vi "Cryo Sep Front Panel.vi"() -> ()   [LabVIEW 2019, in "Results.lvlib" / "Cryo Sep Results.lvclass"]
uses:
  Cryo Sep Results.lvclass
  Test Stands/Cryo Sep/Cryo Sep Test Stand.lvclass
panel:
  out "Temp Timeprofiles":waveform(dbl)[](graph) caption="Temperatures"
  out "Tc5":dbl(slide) scale=0.0..100.0
  out "Tc6":dbl(slide) scale=0.0..100.0
  out "Tc7":dbl(slide) scale=0.0..100.0
  out "Tc8":dbl(slide) scale=0.0..100.0
  out "Tc9":dbl(slide) scale=0.0..100.0
  out "Tc10":dbl(slide) scale=0.0..100.0
  out "Tc11":dbl(slide) scale=0.0..100.0
  out "Tc12":dbl(slide) scale=0.0..100.0
  out "Tc4":dbl(slide) scale=0.0..100.0
  out "Tc4A":dbl(slide) scale=0.0..100.0
  out "Tc4B":dbl(slide) scale=0.0..100.0
  out "Tc4C":dbl(slide) scale=0.0..100.0
  out "Tc2":dbl(slide) scale=0.0..100.0
  out "Tc3":dbl(slide) scale=0.0..100.0
  out "Tc1":dbl(slide) scale=0.0..100.0
  out "Tc0":dbl(slide) max=100.0 scale=0.0..100.0
  out "Tin1":dbl(slide) scale=0.0..100.0
  out "Pressure (abs)":dbl format="%#.2f"
  out "Flow":dbl format="%#.2f"
  out "Tin0":dbl(slide) scale=0.0..100.0
  # "Cryogenic Separator"
  # "l/min (n)"
  # "bar"
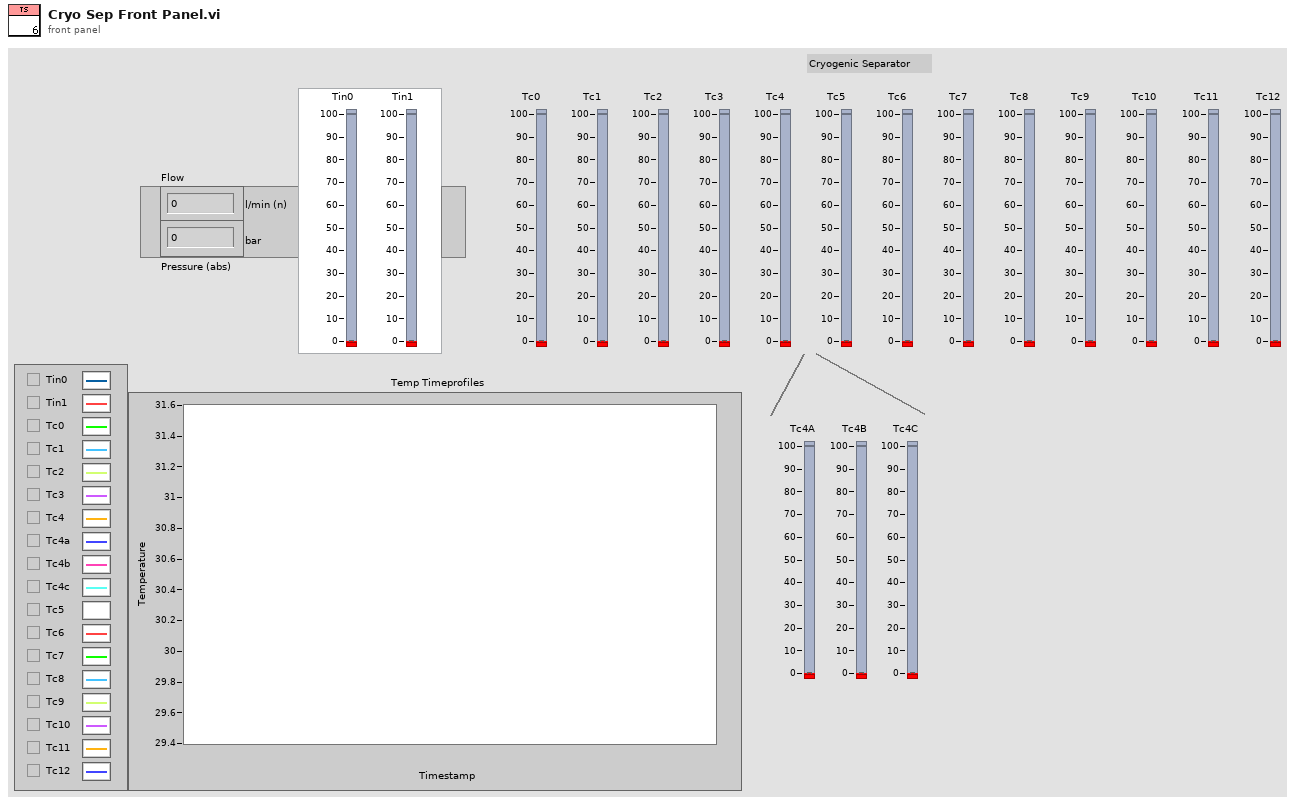
[diagram p1: front panel]
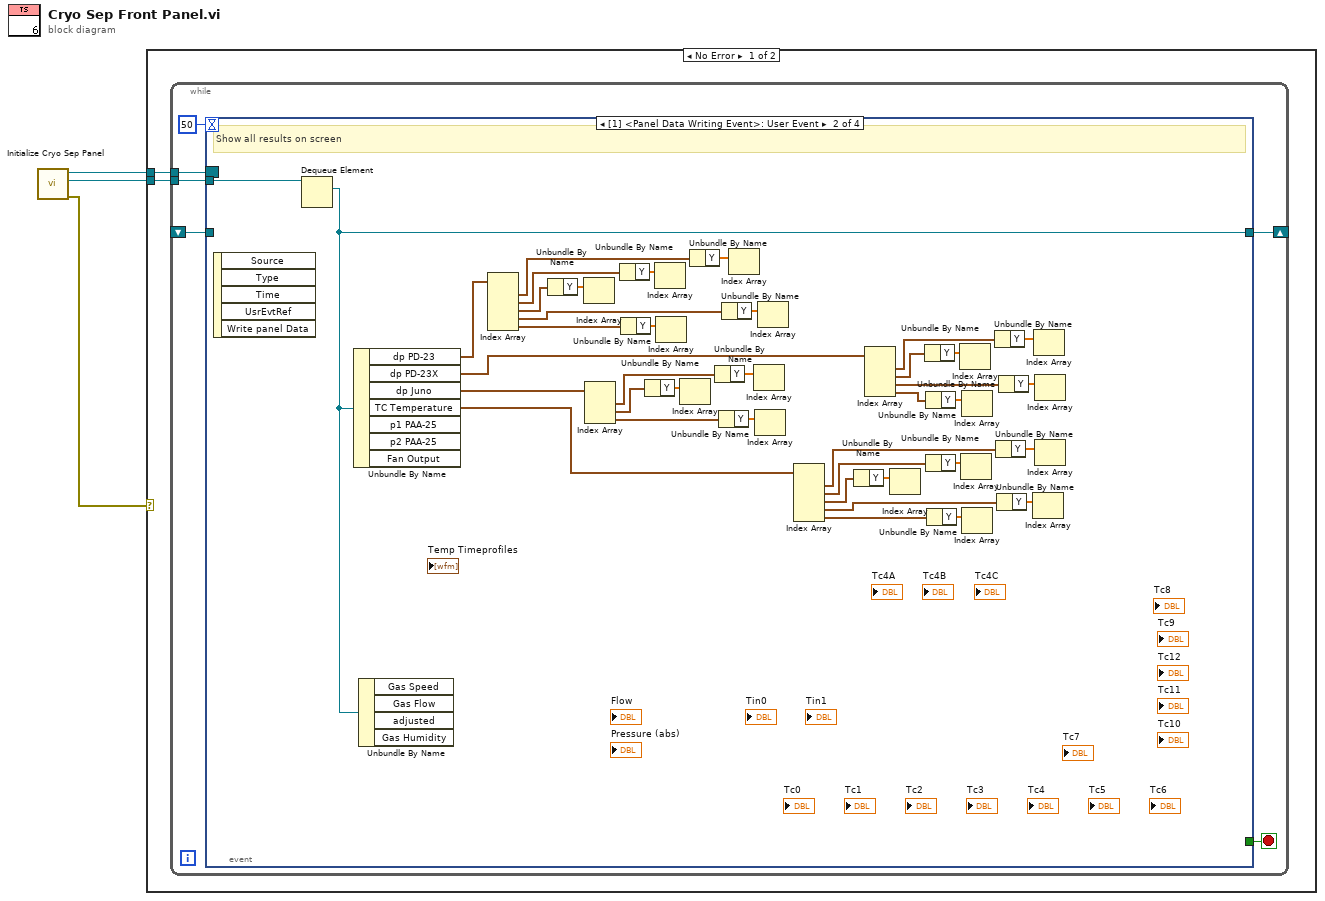
[diagram p0: block diagram]
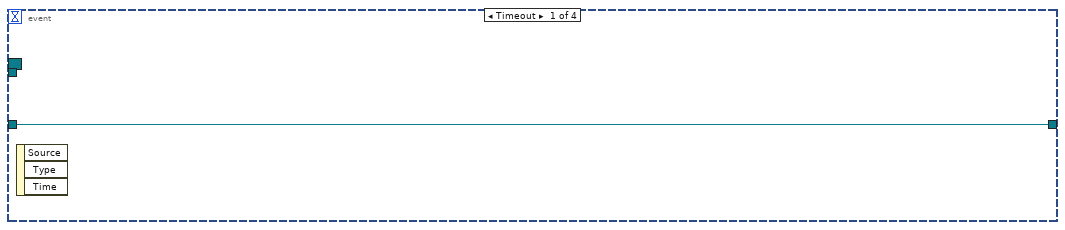
[diagram p2: hidden frame]
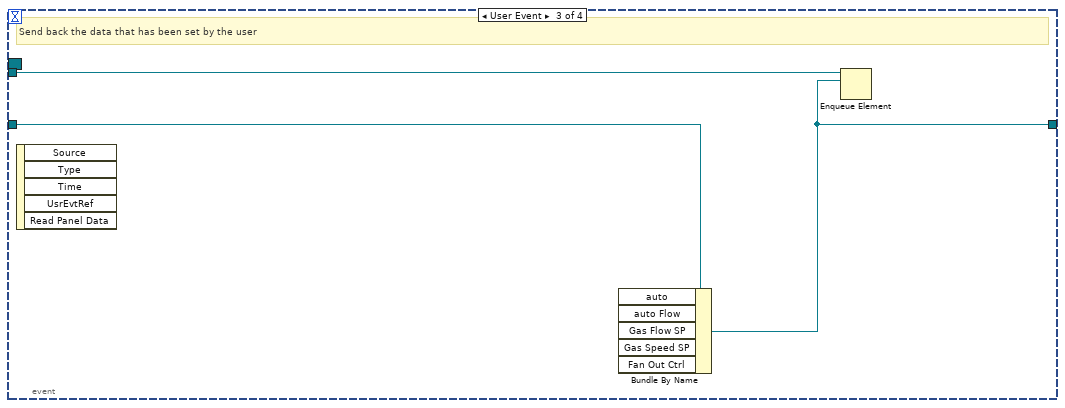
[diagram p3: hidden frame]
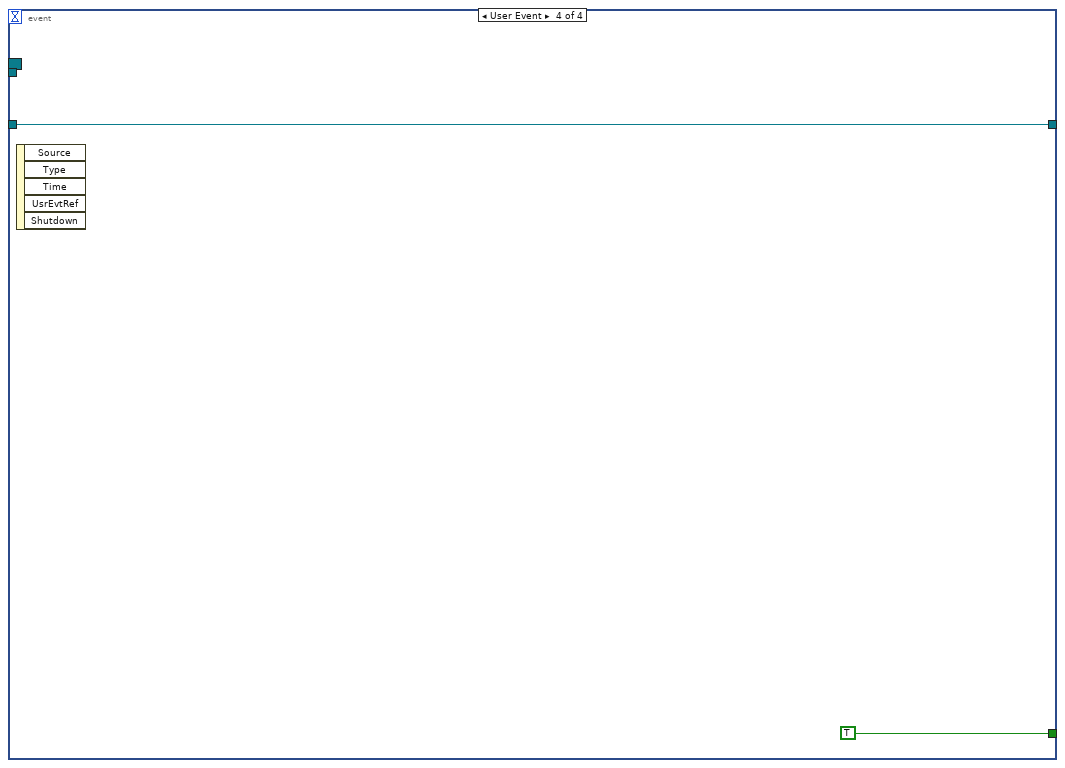
[diagram p4: hidden frame]
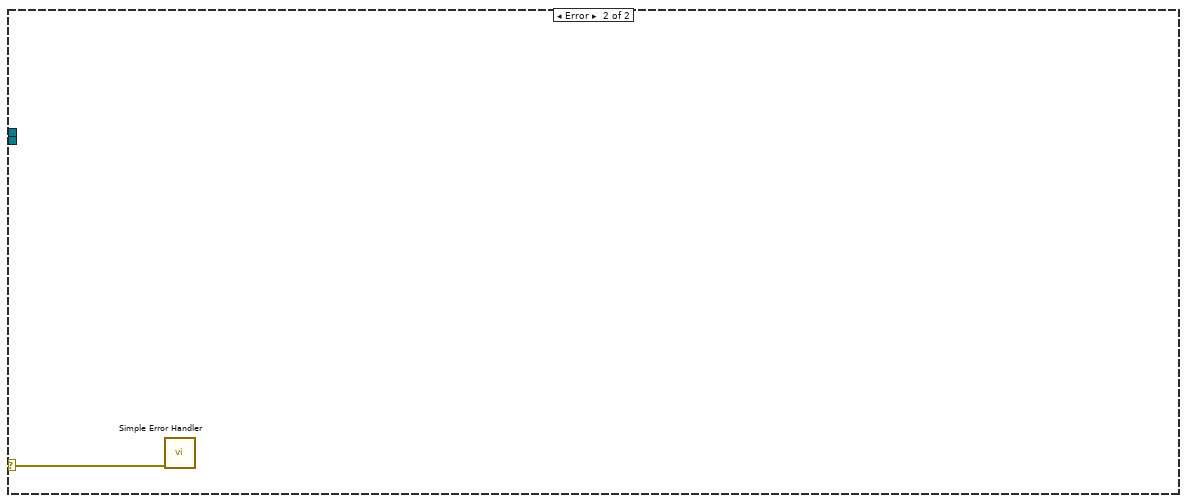
[diagram p5: hidden frame]
diagram:
  n1 = call "Initialize Cryo Sep Panel.vi"() -> ("error out"=w3:errorcluster, "Cryo Sep Results queue out"=w1:refnum<queue>, "Event Registration Refnum"=w2:refnum<event-registration>)  [unwired: 9 in]
  n2 = case shown="No Error" w3 {
    selector: w3 -> [_ w77]
    tunnel: w2 -> [w5 _]
    tunnel: w1 -> [w4 _]
    frame No Error {
      n3 = while {
        tunnel: w5 -> [w10]
        tunnel: w4 -> [w9]
        shift-right: [w7] -> _
        shift-left: _ -> [w6]
        stop <- w11 stop-if-true
        n4 = event shown="[1] <Panel Data Writing Event>: User Event" {
          selector: w10 -> [_ _ _ _]
          dyn-events: _ -> [_ _ _ _]
          timeout: 50 -> [_ _ _ _]
          tunnel: [_ _ _ TRUE] -> w11
          tunnel: w9 -> [_ w66 w74 _]
          tunnel: [w12 w53 w72 w75] -> w7
          tunnel: w6 -> [w12 _ w73 w75]
          event Timeout {
            n5 = event-data() -> ()  [unwired: 1 in, 3 out]
          }
          event User Event {
            # "Show all results on screen"
            n6 = event-data() -> ()  [unwired: 1 in, 5 out]
            n7 = Dequeue Element(queue=w66) -> (element=w53:refnum<class "Cryo Sep Results.lvclass">)  [unwired: 2 in, 3 out]
            n8 = Unbundle By Name(w53) -> ("dp PD-23"=w35:waveform(dbl)[], "dp PD-23X"=w24:waveform(dbl)[], "dp Juno"=w16:waveform(dbl)[], "TC Temperature"=w37:waveform(dbl)[], "p1 PAA-25"=w14:dbl, "p2 PAA-25"=w13:dbl, "Fan Output"=w15:dbl)
            n9 = Unbundle By Name(w53) -> ("Gas Speed"=w52:dbl, "Gas Flow"=w51:dbl, "adjusted"=w50:bool, "Gas Humidity"=w36:dbl)
            n10 = Index Array(array=w35) -> (element #1=w65:waveform(dbl), element #2=w63:waveform(dbl), element #3=w61:waveform(dbl), element #4=w59:waveform(dbl), element #5=w57:waveform(dbl))  [unwired: 5 in]
            n11 = Unbundle By Name(w61) -> ("Y"=w60:dbl[])
            n12 = Index Array(array=w60) -> (element=w55:dbl)  [unwired: 1 in]
            n13 = Index Array(array=w16) -> (element #1=w23:waveform(dbl), element #2=w21:waveform(dbl), element #3=w19:waveform(dbl))  [unwired: 3 in]
            n14 = Unbundle By Name(w63) -> ("Y"=w62:dbl[])
            n15 = Unbundle By Name(w57) -> ("Y"=w56:dbl[])
            n16 = Unbundle By Name(w21) -> ("Y"=w20:dbl[])
            n17 = Index Array(array=w62) -> ()  [unwired: 1 in, 1 out]
            n18 = Index Array(array=w56) -> ()  [unwired: 1 in, 1 out]
            n19 = Index Array(array=w20) -> ()  [unwired: 1 in, 1 out]
            n20 = Unbundle By Name(w65) -> ("Y"=w64:dbl[])
            n21 = Unbundle By Name(w23) -> ("Y"=w22:dbl[])
            n22 = Unbundle By Name(w19) -> ("Y"=w18:dbl[])
            n23 = Unbundle By Name(w59) -> ("Y"=w58:dbl[])
            n24 = Index Array(array=w64) -> ()  [unwired: 1 in, 1 out]
            n25 = Index Array(array=w22) -> ()  [unwired: 1 in, 1 out]
            n26 = Index Array(array=w18) -> (element=w17:dbl)  [unwired: 1 in]
            n27 = Index Array(array=w58) -> (element=w54:dbl)  [unwired: 1 in]
            n28 = Index Array(array=w37) -> (element #1=w38:waveform(dbl), element #2=w40:waveform(dbl), element #3=w42:waveform(dbl), element #4=w44:waveform(dbl), element #5=w46:waveform(dbl))  [unwired: 5 in]
            n29 = Unbundle By Name(w42) -> ("Y"=w43:dbl[])
            n30 = Index Array(array=w24) -> (element #1=w25:waveform(dbl), element #2=w27:waveform(dbl), element #3=w29:waveform(dbl), element #4=w31:waveform(dbl))  [unwired: 4 in]
            n31 = Index Array(array=w43) -> (element=w48:dbl)  [unwired: 1 in]
            n32 = Unbundle By Name(w27) -> ("Y"=w28:dbl[])
            n33 = Unbundle By Name(w31) -> ("Y"=w32:dbl[])
            n34 = Unbundle By Name(w40) -> ("Y"=w41:dbl[])
            n35 = Unbundle By Name(w46) -> ("Y"=w47:dbl[])
            n36 = Index Array(array=w28) -> ()  [unwired: 1 in, 1 out]
            n37 = Index Array(array=w41) -> ()  [unwired: 1 in, 1 out]
            n38 = Index Array(array=w32) -> (element=w34:dbl)  [unwired: 1 in]
            n39 = Index Array(array=w47) -> ()  [unwired: 1 in, 1 out]
            n40 = Unbundle By Name(w25) -> ("Y"=w26:dbl[])
            n41 = Unbundle By Name(w38) -> ("Y"=w39:dbl[])
            n42 = Unbundle By Name(w44) -> ("Y"=w45:dbl[])
            n43 = Unbundle By Name(w29) -> ("Y"=w30:dbl[])
            n44 = Index Array(array=w45) -> (element=w49:dbl)  [unwired: 1 in]
            n45 = Index Array(array=w26) -> ()  [unwired: 1 in, 1 out]
            n46 = Index Array(array=w30) -> (element=w33:dbl)  [unwired: 1 in]
            n47 = Index Array(array=w39) -> ()  [unwired: 1 in, 1 out]
          }
          event User Event {
            # "Send back the data that has been set by the user"
            n48 = event-data() -> ()  [unwired: 1 in, 5 out]
            n49 = Bundle By Name(cluster=w73) -> (w72:refnum<class "Cryo Sep Results.lvclass">, "auto"=w71:bool, "auto Flow"=w70:bool, "Gas Flow SP"=w69:dbl, "Gas Speed SP"=w68:dbl, "Fan Out Ctrl"=w67:dbl)
            n50 = Enqueue Element(queue=w74, element=w72) -> ()  [unwired: 2 in, 3 out]
          }
          event User Event {
            n51 = event-data() -> ()  [unwired: 1 in, 5 out]
          }
        }
      }
    }
    frame Error {
      n52 = call <vilib>:"Simple Error Handler.vi"("error in (no error)"=w77) -> ()  [unwired: 4 in, 5 out]
    }
  }
